vi "Write.vi"(8 "error in (no error)":errorcluster, 10 "Boolean":bool, 11 "Boolean in":refnum<class "FPGA-Bus_Boolean.lvclass">) -> (0 "error out":errorcluster, 3 "Boolean out":refnum<class "FPGA-Bus_Boolean.lvclass">)   [LabVIEW 2021, in "FPGA-Bus_Boolean.lvclass"]
uses:
  FPGA-Bus_Boolean.lvclass
  FPGA-Bus_Boolean.lvclass/FPGA-Bus_Boolean.ctl
  <vilib>/Utility/error.llb/Error Cluster From Error Code.vi
  <vilib>/rvi/errors/niLvFpgaAdjustHostInterfaceError.vi
  <vilib>/rvi/interface/nirviReadWriteControl/nirviReadWriteControl.xnode
  NiFpgaLv.dll
  <vilib>/rvi/interface/Simulation/niFpgaSimulationCallBeginRW.vi
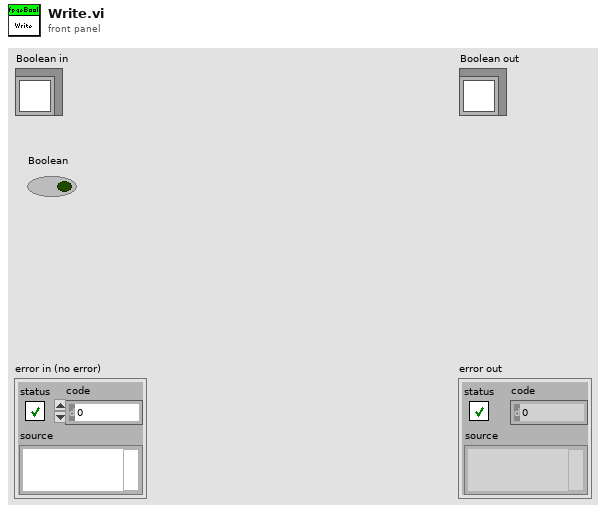
[diagram p1: front panel]
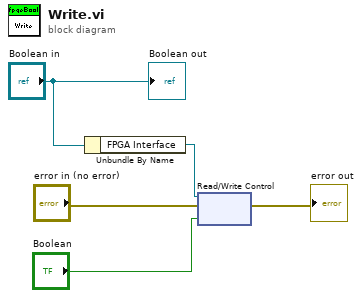
[diagram p0: block diagram]
diagram:
  n1 = Unbundle By Name("Boolean in") -> ("FPGA Interface"=w3:refnum<k20>)
  n2 = xnode "Read/Write Control"("FPGA VI Reference In"=w3, "error in"="error in (no error)", "Value"="Boolean") -> ("error out"=→"error out":errorcluster)  [unwired: 1 out]
  "Boolean out" <- "Boolean in"
